vi "PIDTEMPtest3.vi"() -> ()   [LabVIEW 2015]
uses:
  <vilib>/DAQmx/write.llb/DAQmx Write (Digital 1D Bool NChan 1Samp 1Line).vi
  <vilib>/DAQmx/write.llb/DAQmx Write (Digital Bool 1Line 1Point).vi
  <vilib>/DAQmx/read.llb/DAQmx Read (Analog 1D Wfm NChan 1Samp).vi
  <vilib>/Analysis/baseanly.llb/Mean (DBL).vi
  <vilib>/DAQmx/miscellaneous.llb/DAQmx Fill In Error Info.vi
  <vilib>/Analysis/NI_AALBase.lvlib
  <vilib>/addons/control/pid/NI_PID_autopid.lvlib
panel:
  in  "Heater On/Off":bool
  in  "Manual Control":bool
  out "Control Value":dbl
  in  "setpoint in C":dbl format="%.2f"
  in  "reinitialize? (F)":bool
  in  "autotune? (F)":bool
  out "PID gains out":T1={"proportional gain (Kc)"=1.0, "integral time (Ti, min)"=0.01, "derivative time (Td, min)"=0.0} {"derivative time (Td, min)" format="%.3f"; "integral time (Ti, min)" format="%.3f"; "proportional gain (Kc)" format="%.3f"}
  in  "PID gains":T1={"proportional gain (Kc)"=1.0, "integral time (Ti, min)"=0.01, "derivative time (Td, min)"=0.0} {"derivative time (Td, min)" format="%.3f"; "integral time (Ti, min)" format="%.3f"; "proportional gain (Kc)" format="%.3f"}
  in  "autotuning parameters":T2={"controller type"=1, "relay cycles"=3, "relay amplitude"=1.0, "control specification"=2, "PV noise level"=0.1} {"PV noise level" format="%.2f"; "control specification" items=["normal", "fast", "slow"]; "relay amplitude" format="%.2f"; "controller type" items=["PID", "PI", "P"]}
  in  "stop":bool
  out "Temp":dbl
  out "Temp Chart 2":waveform(dbl)(graph)
  out "Temp Chart":waveform(dbl)(graph)
  out "Temp(C)":dbl(slide) scale=-10.0..100.0
  out "Temperature (Celcius)":dbl format="%#.1g"
  out "Voltage Reading(Temp)":dbl format="%#_13g"
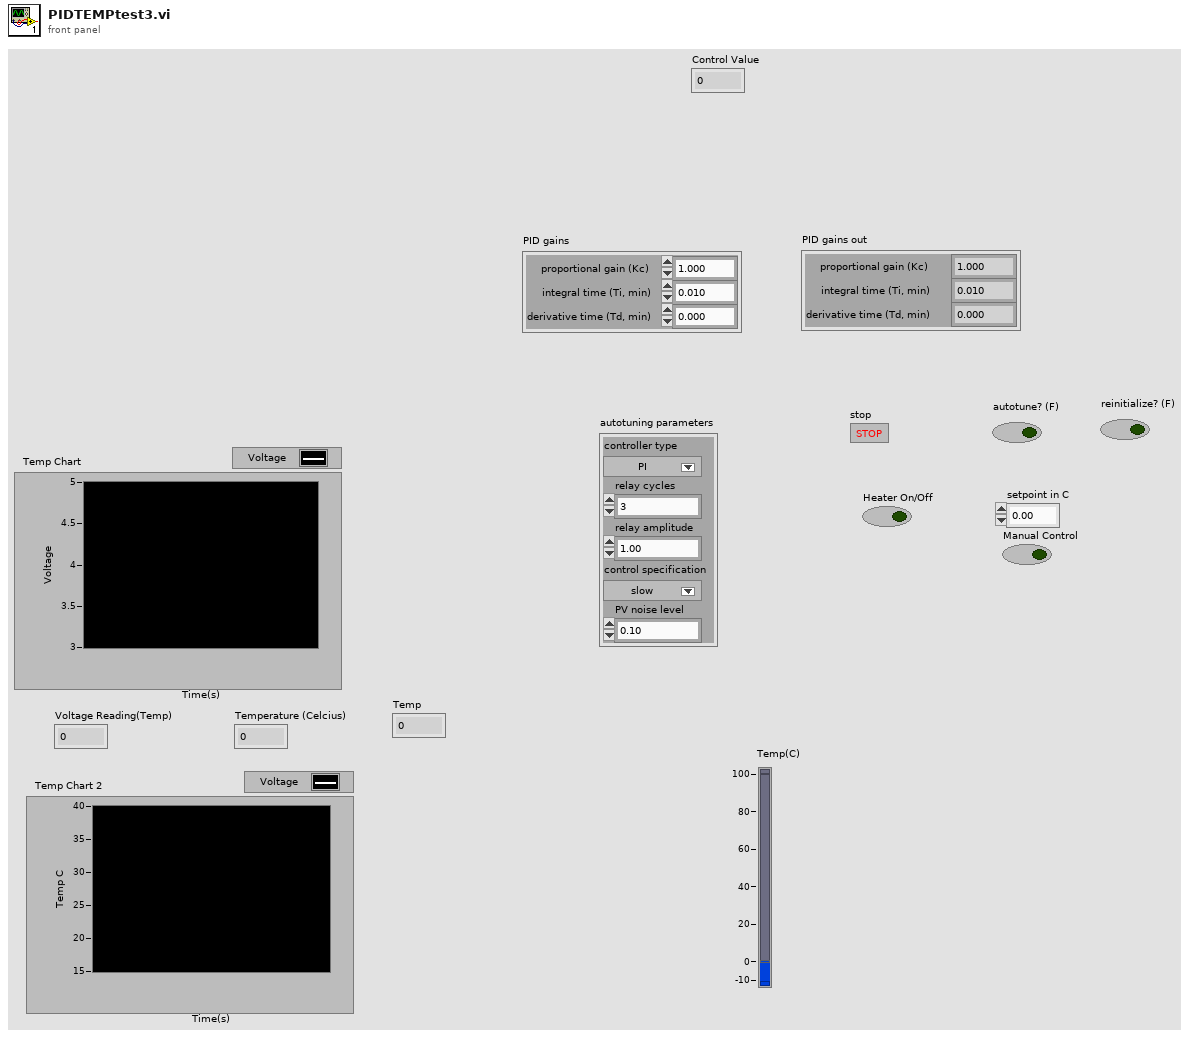
[diagram p1: front panel]
types:
  T1 = cluster{"proportional gain (Kc)":dbl, "integral time (Ti, min)":dbl, "derivative time (Td, min)":dbl}
  T2 = cluster{"controller type":u16, "relay cycles":i32, "relay amplitude":dbl, "control specification":u16, "PV noise level":dbl}
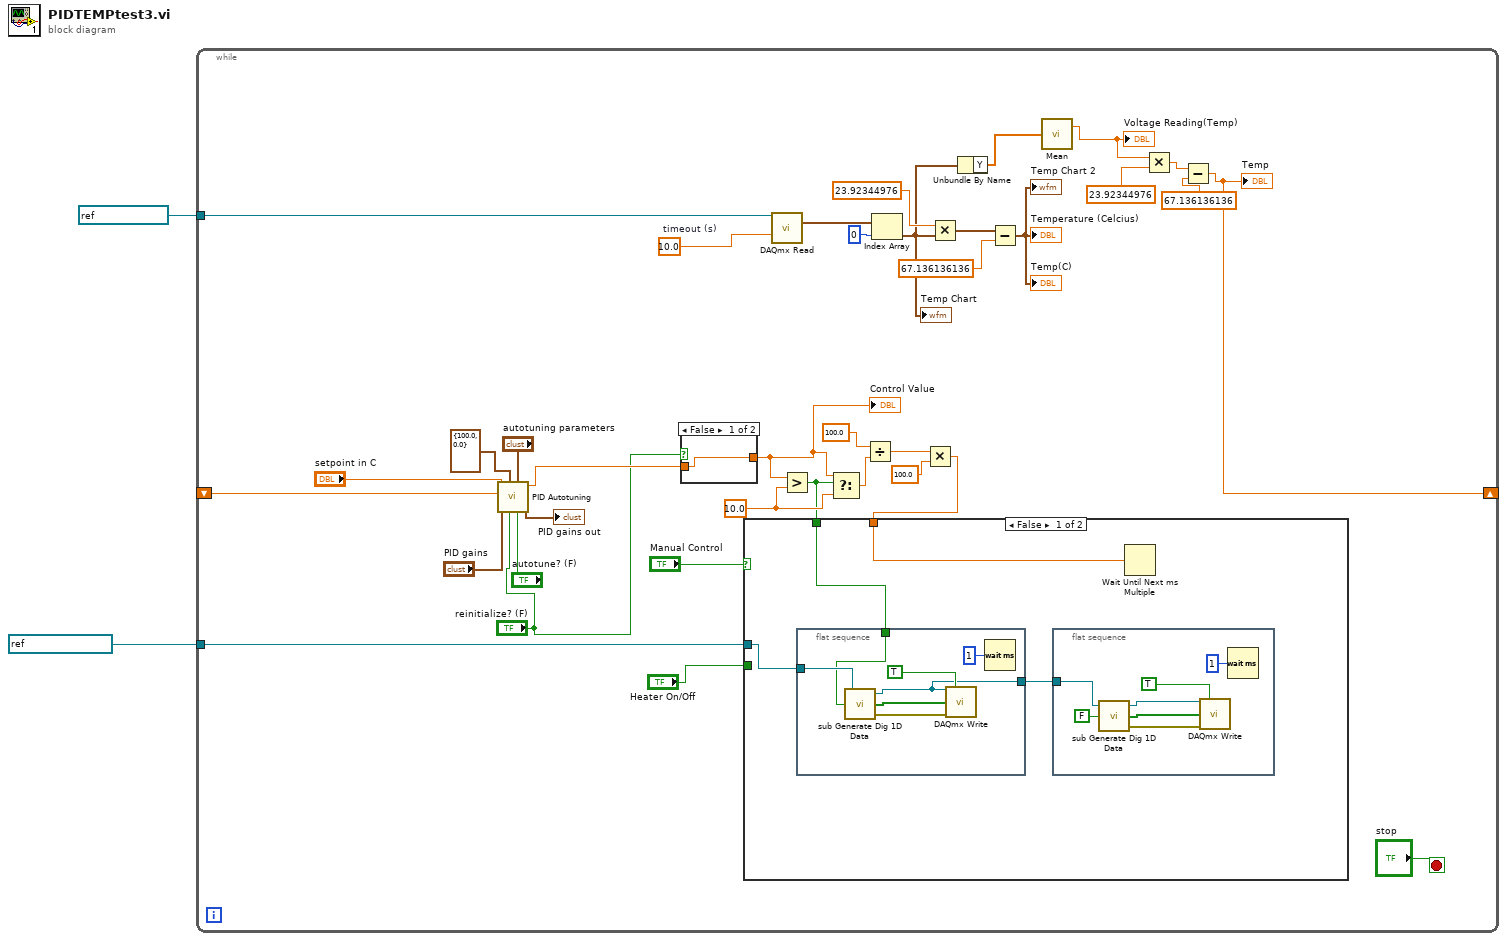
[diagram p0: block diagram]
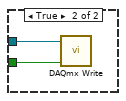
[diagram p2: hidden frame]
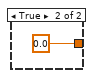
[diagram p3: hidden frame]
diagram:
  n1 = while {
    tunnel: refnum<k21> "AnalogInA0" -> [w25]
    shift-right: [w23] -> _
    shift-left: _ -> [w18]
    tunnel: refnum<k21> "YellowdigOUT" -> [w12]
    stop <- "stop" stop-if-true
    w4 = 10.0 ("f")
    w38 = 10.0  # timeout (s)
    n2 = call <vilib>:"PID Autotuning.vi"("autotune? (F)"="autotune? (F)", "autotuning parameters"="autotuning parameters", "reinitialize? (F)"="reinitialize? (F)", "output range"=cluster{"output high":dbl, "output low":dbl} {"output high"=100.0, "output low"=0.0}, "PID gains"="PID gains", "process variable"=w18, "setpoint"="setpoint in C") -> ("PID gains out"=→"PID gains out":T1, "output"=w16:dbl)  [unwired: 1 in, 2 out]
    n3 = case shown="False" "reinitialize? (F)" {
      tunnel: [w59 0.0] -> w5
      tunnel: w16 -> [w59 _]
      frame False {
      }
      frame True {
      }
    }
    "Control Value" <- w5
    n4 = call-poly <vilib>:"DAQmx Read.vi"("task/channels in"=w25, "timeout"=w38) -> ("data"=w33:waveform(dbl)[])  [unwired: 11 in, 2 out]
    n5 = Greater?(x=w5, y=w4) -> (0:w3:bool)
    n6 = Select(t=w5, s=w3, f=w4) -> (s? t:f=w6:dbl)
    n7 = Divide(x=100.0, y=w6) -> (x/y=w9:dbl)
    n8 = Index Array(array=w33, index=0) -> (element=w31:waveform(dbl))
    "Temp Chart" <- w31
    n9 = Multiply(x=w9, y=100.0) -> (x*y=w7:dbl)
    n10 = case shown="False" "Manual Control" {
      tunnel: w12 -> [w41 w58]
      tunnel: "Heater On/Off" -> [_ w57]
      tunnel: w7 -> [w40 _]
      tunnel: w3 -> [w39 _]
      frame False {
        n11 = flat-sequence {
          tunnel: w41 -> [w53]
          tunnel: [w52] -> w42
          tunnel: w39 -> [w51]
          frame #0 {
            n12 = call <vilib>:"sub Generate Dig 1D Data.vi"("initial value"=w51, "task in"=w53) -> ("error out"=w55:errorcluster, "Data"=w56:bool[], "task out"=w52:refnum<k21>)  [unwired: 1 in]
            n13 = call-poly <vilib>:"DAQmx Write.vi"("task/channels in"=w52, "auto start"=TRUE, "data"=w56, "error in"=w55) -> ()  [unwired: 9 in, 3 out]
            n14 = Wait (ms)(milliseconds to wait=u32 1) -> ()  [unwired: 1 out]
          }
        }
        n15 = flat-sequence {
          tunnel: w42 -> [w44]
          frame #0 {
            n16 = call <vilib>:"sub Generate Dig 1D Data.vi"("initial value"=FALSE, "task in"=w44) -> ("error out"=w48:errorcluster, "Data"=w46:bool[], "task out"=w47:refnum<k21>)  [unwired: 1 in]
            n17 = call-poly <vilib>:"DAQmx Write.vi"("task/channels in"=w47, "auto start"=TRUE, "data"=w46, "error in"=w48) -> ()  [unwired: 9 in, 3 out]
            n18 = Wait (ms)(milliseconds to wait=u32 1) -> ()  [unwired: 1 out]
          }
        }
        n19 = Wait Until Next ms Multiple(millisecond multiple=w40) -> ()  [unwired: 1 out]
      }
      frame True {
        n20 = call-poly <vilib>:"DAQmx Write.vi"("task/channels in"=w58, "data"=w57) -> ()  [unwired: 11 in, 3 out]
      }
    }
    n21 = Multiply(x=23.92344976, y=w31) -> (x*y=w36:waveform(dbl))
    n22 = Unbundle By Name(w31) -> ("Y"=w30:dbl[])
    n23 = Subtract(x=w36, y=67.136136136) -> (x-y=→"Temperature (Celcius)" →"Temp(C)" →"Temp Chart 2":waveform(dbl))
    n24 = call-poly <vilib>:"Mean.vi"("X"=w30) -> ("mean"=w29:dbl)  [unwired: 1 out]
    "Voltage Reading(Temp)" <- w29
    n25 = Multiply(x=w29, y=23.92344976) -> (x*y=w28:dbl)
    n26 = Subtract(x=w28, y=67.136136136) -> (x-y=w23:dbl)
    "Temp" <- w23
  }
